vi "getChannel_name.vi"(8 "error in (no error)":errorcluster, 11 "Channel.lvclass in":refnum<class "Channel.lvclass">) -> (0 "error out":errorcluster, 2 "channel_name":string, 3 "Channel.lvclass out":refnum<class "Channel.lvclass">)   [LabVIEW 2009, in "Tools.lvlib" / "DatabaseHelpers.lvlib" / "Channel.lvclass"]
uses:
  Channel.lvclass
  Channel.lvclass/Channel.ctl
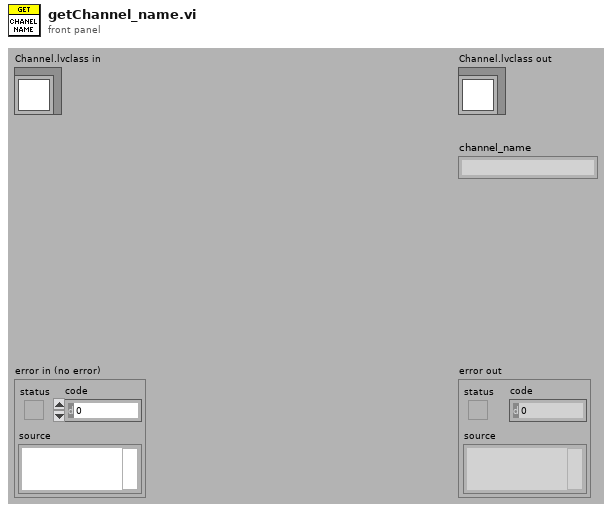
[diagram p1: front panel]
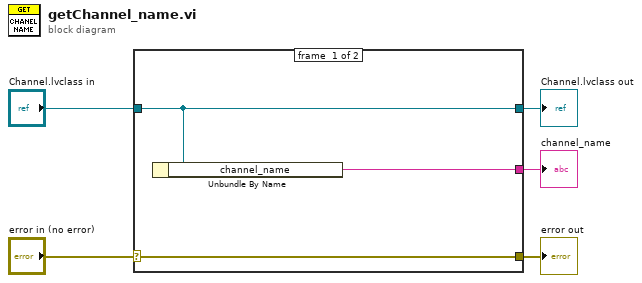
[diagram p0: block diagram]
diagram:
  n1 = case shown="No Error" "error in (no error)" {
    selector: "error in (no error)" -> [w8 w9]
    tunnel: [w8 w9] -> w4
    tunnel: [w7 w10] -> w2
    tunnel: "Channel.lvclass in" -> [w7 w10]
    tunnel: [w6 _] -> w1
    frame #0 {
      n2 = Unbundle By Name(w7) -> ("channel_name"=w6:string)
    }
    frame #1 {
    }
  }
  "error out" <- w4
  "Channel.lvclass out" <- w2
  "channel_name" <- w1
